vi "Main.TestDB.vi"   [LabVIEW 2016]
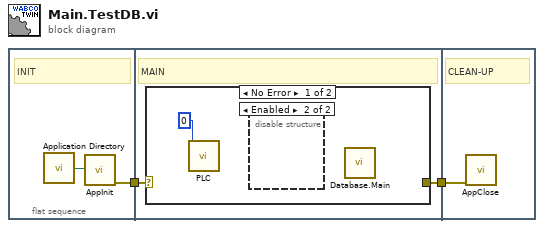
[diagram p0: block diagram]
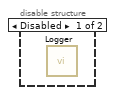
[diagram p2: hidden frame]
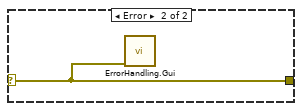
[diagram p3: hidden frame]
diagram:
  n1 = flat-sequence {
    tunnel: [w3] -> w2
    tunnel: w2 -> [w6]
    tunnel: [w5] -> w1
    tunnel: w1 -> [w9]
    frame #0 {
      # "INIT"
      n2 = call <vilib>:"Application Directory.vi"() -> ("Application Directory"=w4:path)
      n3 = call "AppInit.vi"("path"=w4) -> ("error out"=w3:errorcluster)  [unwired: 10 in]
    }
    frame #1 {
      # "MAIN"
      n4 = case shown="No Error" w6 {
        selector: w6 -> [_ w8]
        tunnel: [_ w8] -> w5
        frame No Error {
          n5 = call "PLC.vi"("Idx"=0) -> ()  [unwired: 11 in]
          n6 = disable-structure shown="Enabled" {
            frame Disabled {
              n7 = call "Logger.vi"() -> ()  [unwired: 12 in]
            }
            frame Enabled {
            }
          }
          n8 = call "Database.Main.vi"() -> ()  [unwired: 1 in]
        }
        frame Error {
          n9 = call "ErrorHandling.Gui.vi"("error in (no error)"=w8) -> ()  [unwired: 9 in, 2 out]
        }
      }
    }
    frame #2 {
      # "CLEAN-UP"
      n10 = call "AppClose.vi"("error in (no error)"=w9) -> ()  [unwired: 11 in]
    }
  }
